vi "_FG_save_LV2018.vi"(6 "comment":string, 7 "error in":errorcluster, 8 "add EOL at end ?":bool, 9 "data in":variant, 10 "FG":T1) -> (0 "error IO":errorcluster={"status"=TRUE, "code"=1, "source"="Écrire dans un fichier texte dans _FG_save_LV2018.vi->save_all_parameters.vi->_main_program v5.vi"})   [LabVIEW 2018]
uses:
  enum_fg_save.ctl
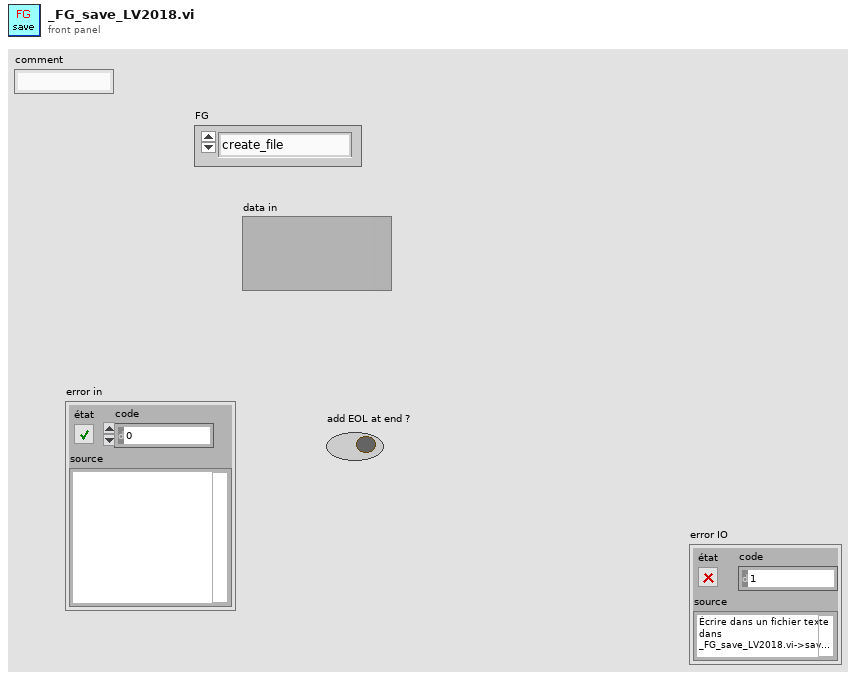
[diagram p1: front panel]
types:
  T1 = typedef "enum_fg_save.ctl" = enum16{"create_file", "w_array_text_inline", "w_text", "w_int", "w_uint", "w_single", "w_array", "w_array_inline", "w_clst_2arrays", "w_clst_3arrays", "w_clst_4arrays", "w_clst_5arrays", "w_clst_6arrays", "w_2Darray", "w_time", "close_file"}
  T2 = enum16{"open", "replace", "create", "open or create", "replace or create", "replace or create with confirmation"}
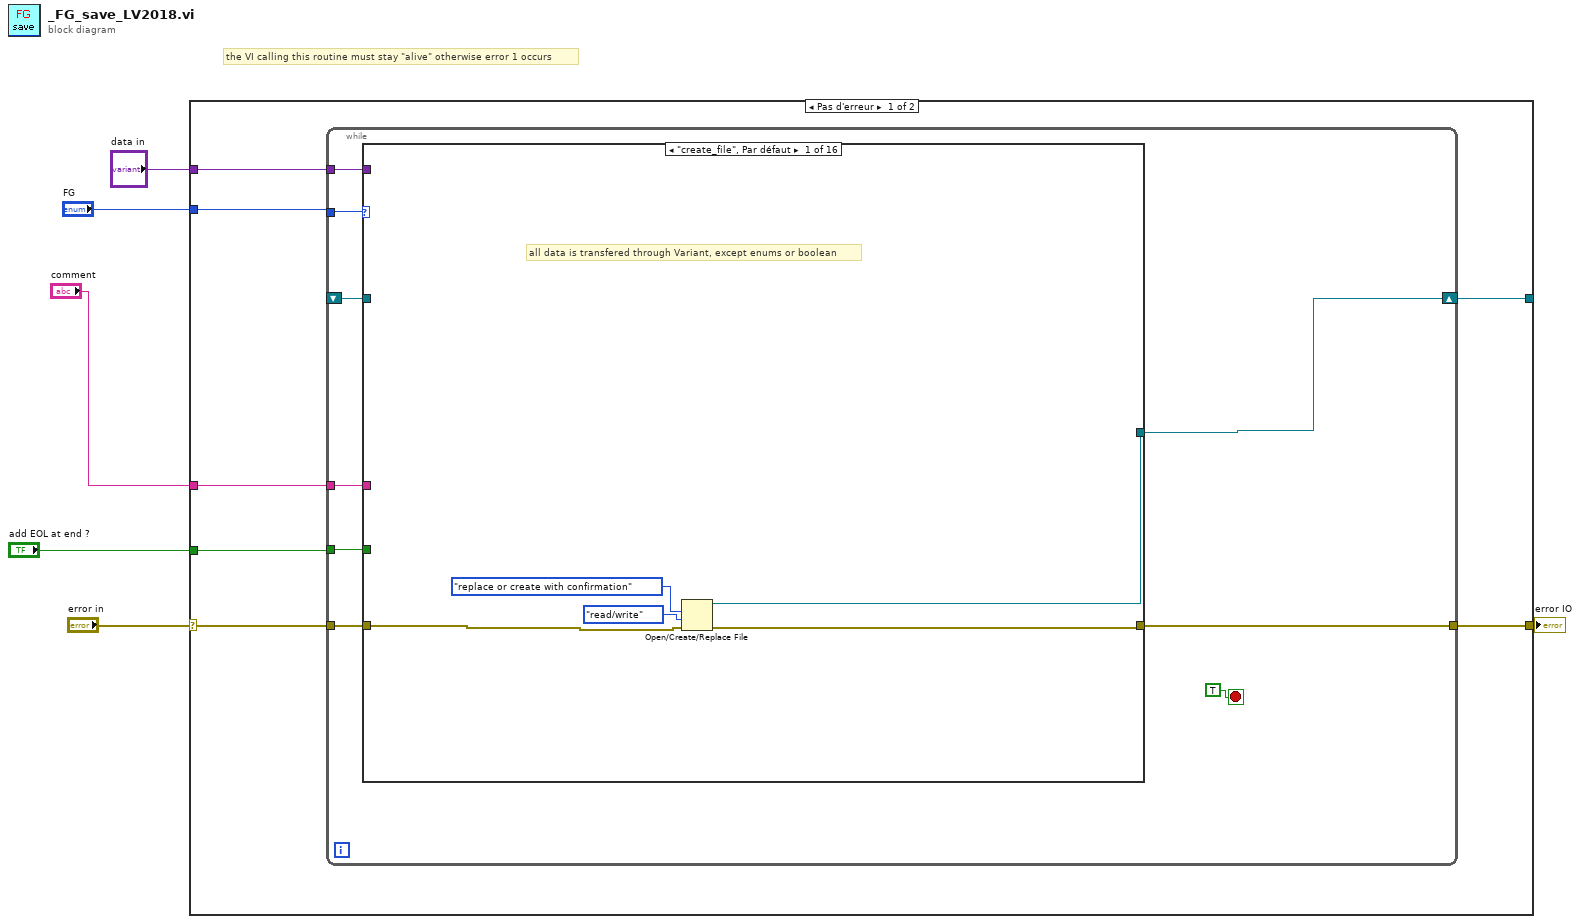
[diagram p0: block diagram]
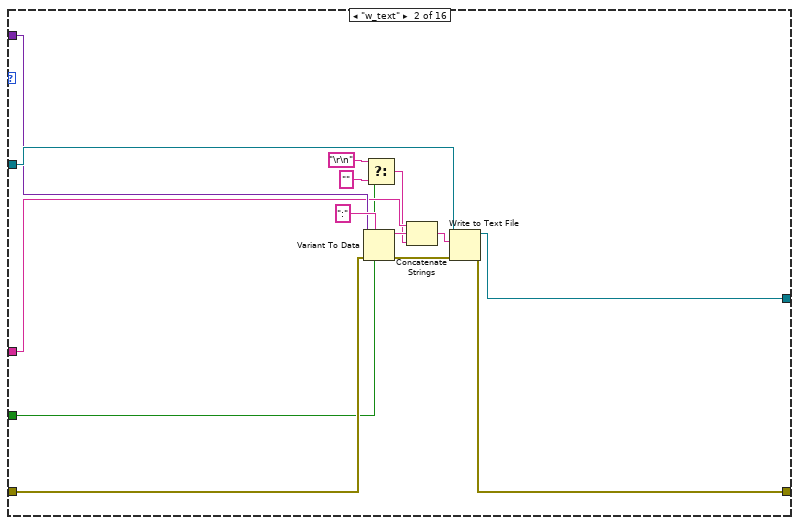
[diagram p2: hidden frame]
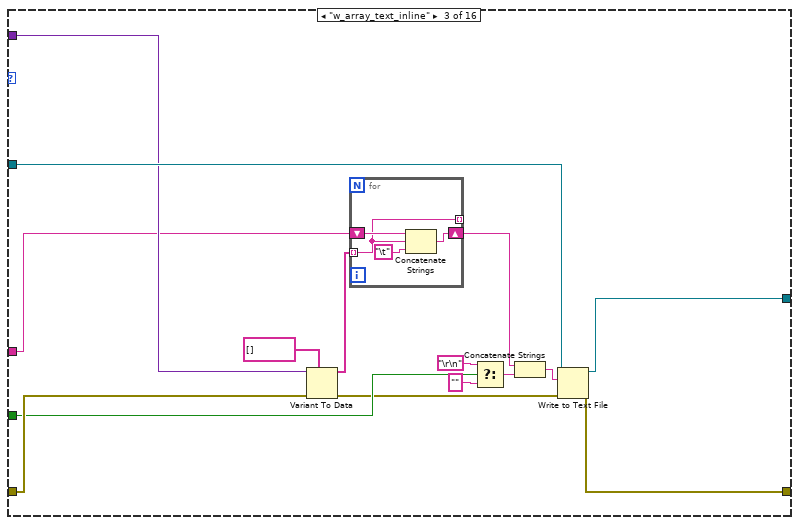
[diagram p3: hidden frame]
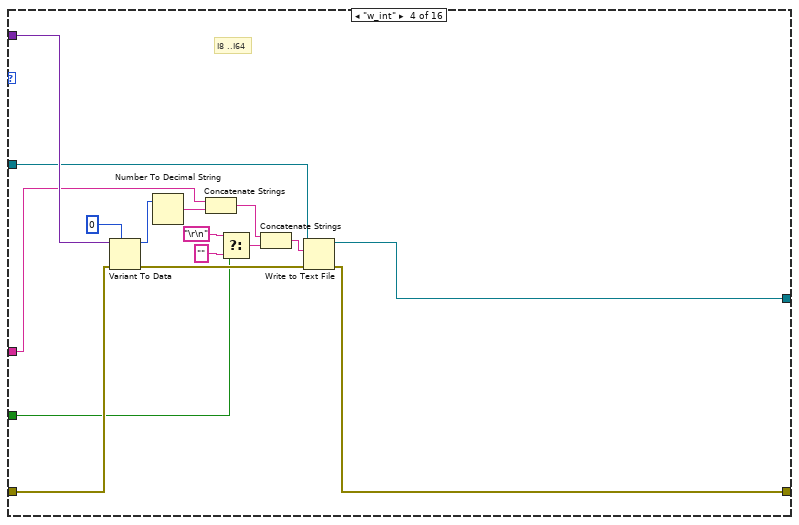
[diagram p4: hidden frame]
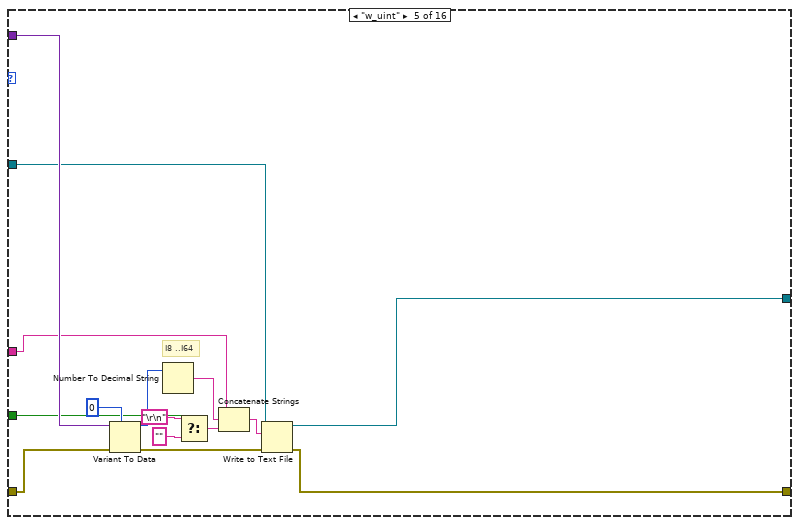
[diagram p5: hidden frame]
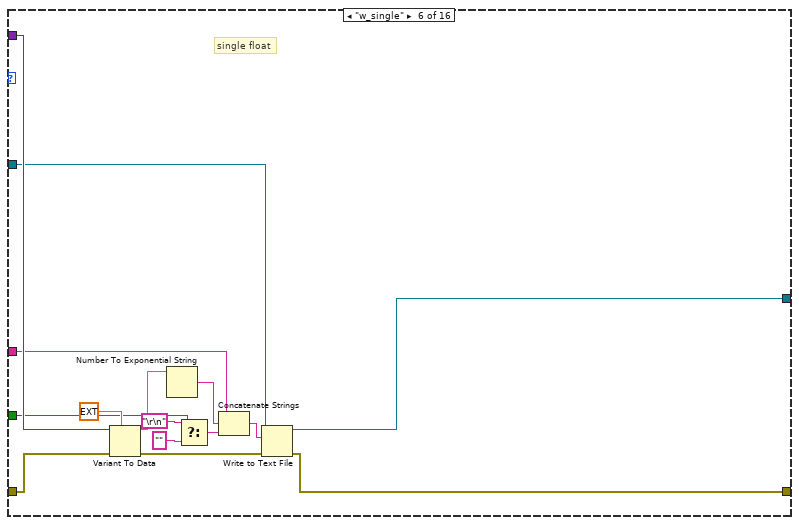
[diagram p6: hidden frame]
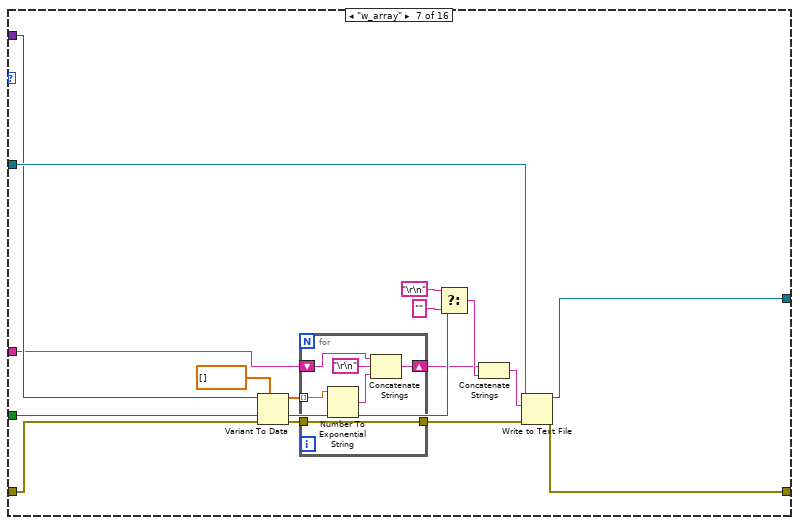
[diagram p7: hidden frame]
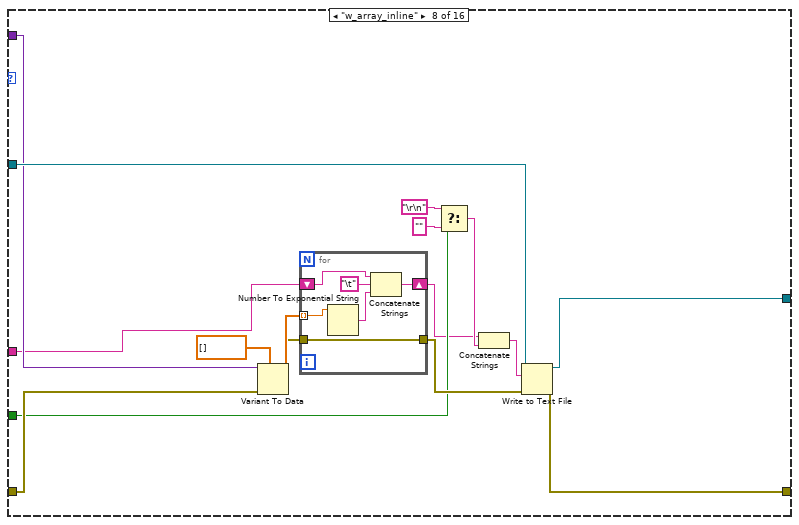
[diagram p8: hidden frame]
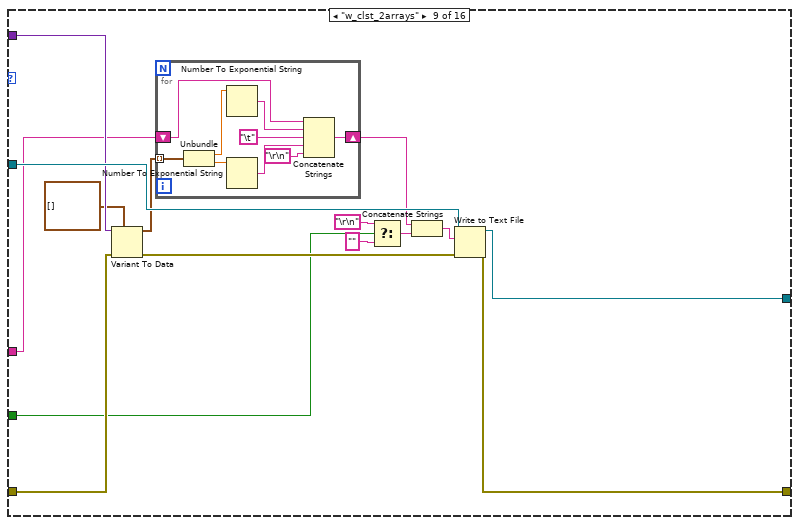
[diagram p9: hidden frame]
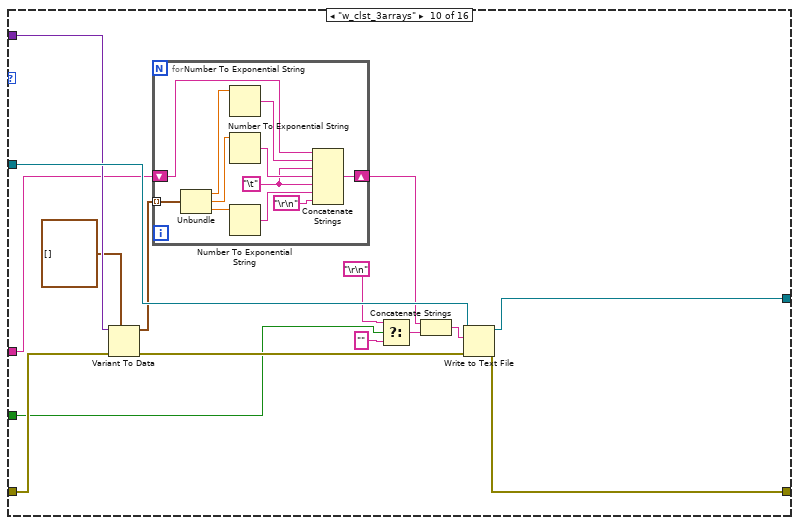
[diagram p10: hidden frame]
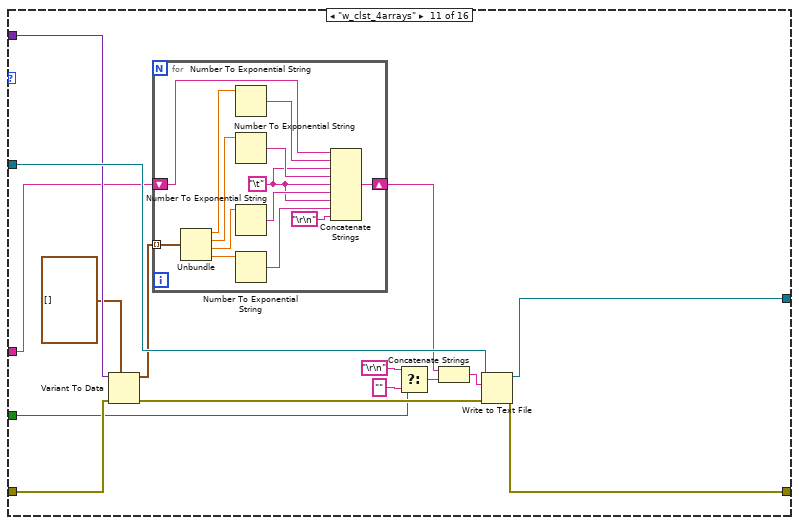
[diagram p11: hidden frame]
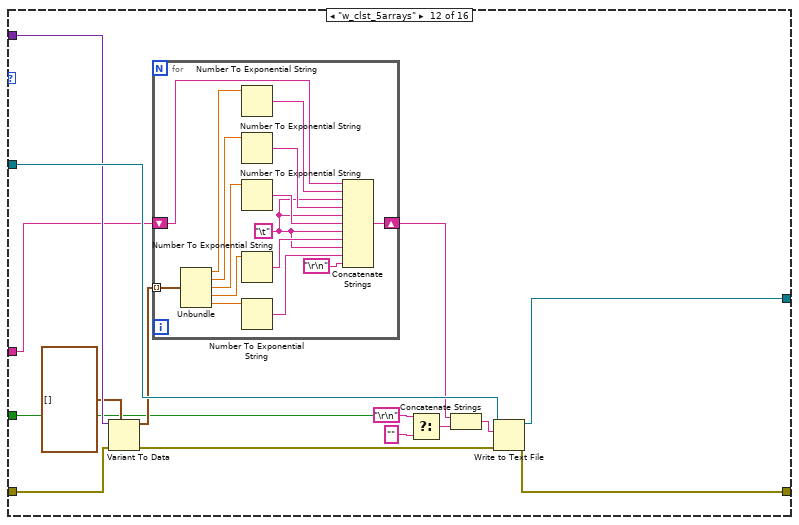
[diagram p12: hidden frame]
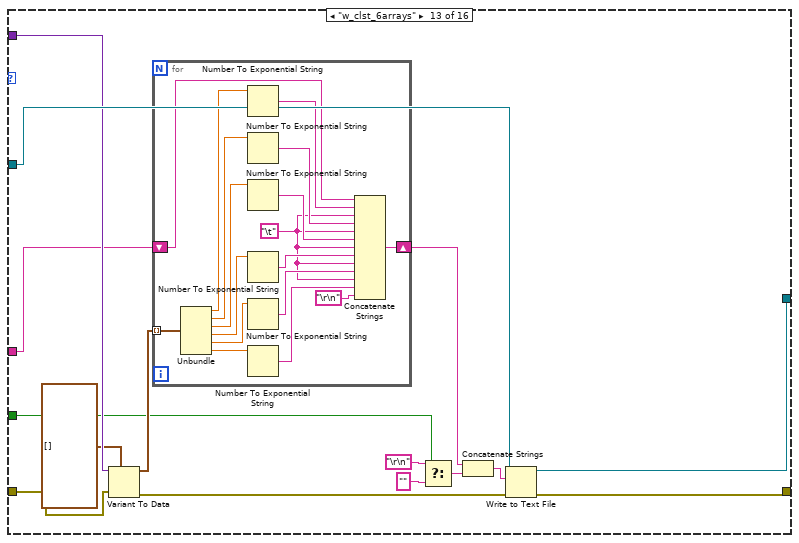
[diagram p13: hidden frame]
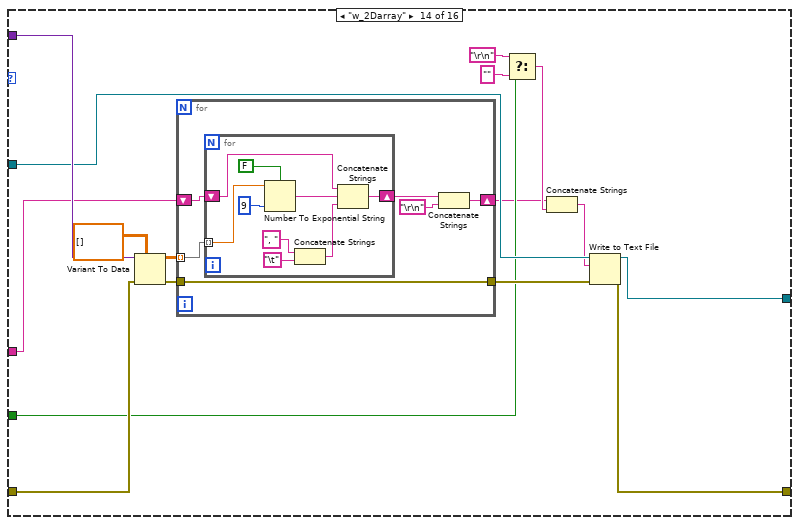
[diagram p14: hidden frame]
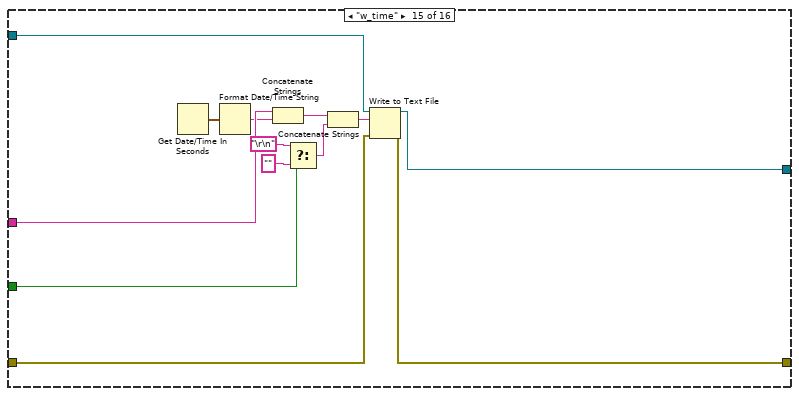
[diagram p15: hidden frame]
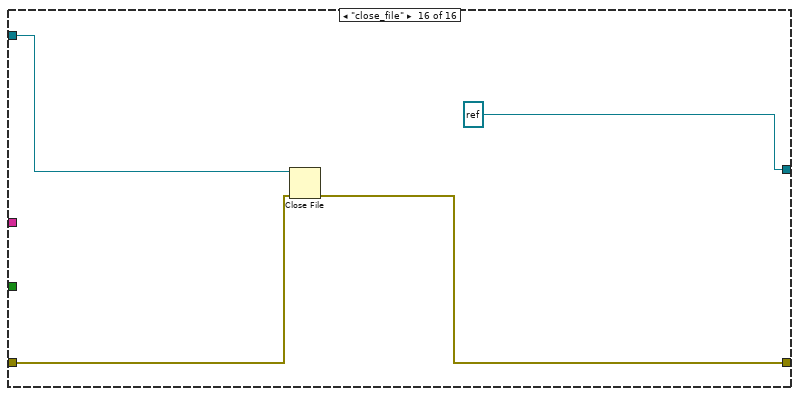
[diagram p16: hidden frame]
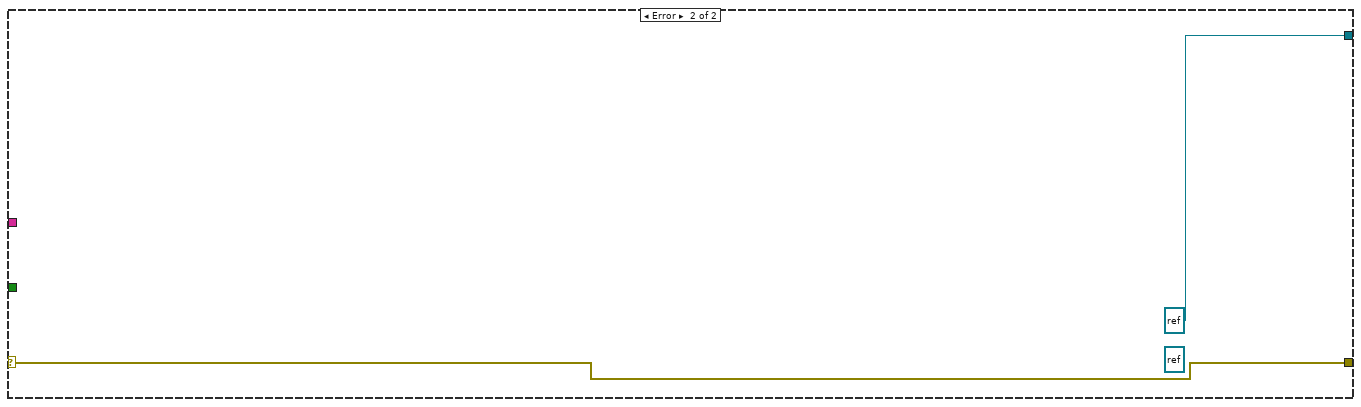
[diagram p17: hidden frame]
diagram:
  # "the VI calling this routine must stay \"alive\" otherwise error 1 occurs"
  n1 = case shown="Pas d'erreur" "error in" {
    selector: "error in" -> [w12 w339]
    tunnel: "FG" -> [w13 _]
    tunnel: [w11 refnum<file> refnum ("refnum out")] -> _
    tunnel: [w10 w339] -> w3
    tunnel: "data in" -> [w9 _]
    tunnel: "comment" -> [w8 _]
    tunnel: "add EOL at end ?" -> [w7 _]
    frame No Error {
      n2 = while {
        tunnel: w13 -> [w21]
        tunnel: w12 -> [w20]
        shift-right: [w15] -> w11
        shift-left: _ -> [w19]
        tunnel: [w14] -> w10
        tunnel: w9 -> [w18]
        tunnel: w8 -> [w17]
        tunnel: w7 -> [w16]
        stop <- TRUE stop-if-true
        n3 = case shown="\"create_file\", Par défaut" w21 {
          tunnel: w20 -> [w25 w36 w52 w74 w89 w104 w115 w137 w159 w183 w209 w237 w267 w304 w333 w335]
          tunnel: [w24 w40 w55 w71 w86 w101 w120 w142 w164 w188 w214 w242 w272 w299 w331 refnum<file> refnum ("refnum out")] -> w15
          tunnel: [w23 w41 w56 w70 w85 w100 w121 w143 w165 w189 w215 w243 w273 w300 w334 w336] -> w14
          tunnel: w19 -> [_ w39 w54 w72 w87 w102 w119 w141 w163 w187 w213 w241 w271 w298 w330 w338]
          tunnel: w18 -> [_ w37 w53 w75 w90 w105 w117 w139 w162 w186 w212 w240 w270 w305 _ _]
          tunnel: w17 -> [_ w35 w49 w68 w83 w98 w113 w135 w157 w181 w207 w235 w265 w297 w329 _]
          tunnel: w16 -> [_ w30 w44 w63 w78 w93 w109 w131 w153 w177 w203 w231 w261 w293 w324 _]
          frame "create_file", Default {
            # "all data is transfered through Variant, except enums or boolean"
            n4 = Open/Create/Replace File(error in=w25, operation (0:open)=T2."replace or create with confirmation" ("opération (0 : open)"), access (0:read/write)=enum16{"read/write", "read-only", "write-only"}."read/write" ("accès (0 : read/write)")) -> (refnum out=w24:refnum<file>, error out=w23:errorcluster)  [unwired: 3 in, 1 out]
          }
          frame "w_text" {
            n5 = Variant To Data(error in=w36, type=":" ("chaîne recherchée"), Variant=w37) -> (data=w34:string, error out=w28:errorcluster)
            n6 = Select(t="\r\n", s=w30, f="" ("cas faux")) -> (s? t:f=w29:string)
            n7 = Concatenate Strings(w35, w34, w29) -> (w33:string)
            n8 = Write to Text File(file (use dialog)=w39, text=w33, error in=w28) -> (refnum out=w40:refnum<file>, error out=w41:errorcluster)  [unwired: 1 in, 1 out]
          }
          frame "w_array_text_inline" {
            n9 = Variant To Data(error in=w52, type=string[] [] ("Tableau"), Variant=w53) -> (data=w50:string[], error out=w42:errorcluster)
            n10 = for {
              tunnel: [w59] -> _ mode=indexing
              tunnel: w50 -> [w59] mode=indexing
              shift-right: [w57] -> w46
              shift-left: w49 -> [w60]
              n11 = Concatenate Strings(w60, w59, "\t") -> (w57:string)
            }
            n12 = Select(t="\r\n", s=w44, f="" ("cas faux")) -> (s? t:f=w45:string)
            n13 = Concatenate Strings(w46, w45) -> (w43:string)
            n14 = Write to Text File(file (use dialog)=w54, text=w43, error in=w42) -> (refnum out=w55:refnum<file>, error out=w56:errorcluster)  [unwired: 1 in, 1 out]
          }
          frame "w_int" {
            # "I8 ..I64"
            n15 = Variant To Data(error in=w74, type=i64 0 ("r * e^(i*thêta)"), Variant=w75) -> (data=w73:i64, error out=w69:errorcluster)
            n16 = Number To Decimal String(number=w73) -> (decimal integer string=w67:string)  [unwired: 1 in]
            n17 = Concatenate Strings(w68, w67) -> (w62:string)
            n18 = Select(t="\r\n", s=w63, f="" ("cas faux")) -> (s? t:f=w64:string)
            n19 = Concatenate Strings(w62, w64) -> (w61:string)
            n20 = Write to Text File(file (use dialog)=w72, text=w61, error in=w69) -> (refnum out=w71:refnum<file>, error out=w70:errorcluster)  [unwired: 1 in, 1 out]
          }
          frame "w_uint" {
            # "I8 ..I64"
            n21 = Variant To Data(error in=w89, type=u64 0 ("r * e^(i*thêta)"), Variant=w90) -> (data=w88:u64, error out=w84:errorcluster)
            n22 = Number To Decimal String(number=w88) -> (decimal integer string=w82:string)  [unwired: 1 in]
            n23 = Select(t="\r\n", s=w78, f="" ("cas faux")) -> (s? t:f=w77:string)
            n24 = Concatenate Strings(w83, w82, w77) -> (w81:string)
            n25 = Write to Text File(file (use dialog)=w87, text=w81, error in=w84) -> (refnum out=w86:refnum<file>, error out=w85:errorcluster)  [unwired: 1 in, 1 out]
          }
          frame "w_single" {
            # "single float"
            n26 = Variant To Data(error in=w104, type=ext 0.0 ("r * e^(i*thêta)"), Variant=w105) -> (data=w103:ext, error out=w99:errorcluster)
            n27 = Number To Exponential String(number=w103) -> (E-format string=w97:string)  [unwired: 3 in]
            n28 = Select(t="\r\n", s=w93, f="" ("cas faux")) -> (s? t:f=w92:string)
            n29 = Concatenate Strings(w98, w97, w92) -> (w96:string)
            n30 = Write to Text File(file (use dialog)=w102, text=w96, error in=w99) -> (refnum out=w101:refnum<file>, error out=w100:errorcluster)  [unwired: 1 in, 1 out]
          }
          frame "w_array" {
            n31 = Variant To Data(error in=w115, type=dbl[] [] ("array 1"), Variant=w117) -> (data=w116:dbl[], error out=w114:errorcluster)
            n32 = for {
              tunnel: w116 -> [w127] mode=indexing
              shift-right: [w128] -> w108
              shift-left: w113 -> [w126]
              tunnel: w114 -> [w123]
              tunnel: [w123] -> w122
              n33 = Number To Exponential String(number=w127) -> (E-format string=w124:string)  [unwired: 3 in]
              n34 = Concatenate Strings(w126, "\r\n", w124) -> (w128:string)
            }
            n35 = Select(t="\r\n", s=w109, f="" ("cas faux")) -> (s? t:f=w110:string)
            n36 = Concatenate Strings(w108, w110) -> (w107:string)
            n37 = Write to Text File(file (use dialog)=w119, text=w107, error in=w122) -> (refnum out=w120:refnum<file>, error out=w121:errorcluster)  [unwired: 1 in, 1 out]
          }
          frame "w_array_inline" {
            n38 = Variant To Data(error in=w137, type=dbl[] [] ("array 1"), Variant=w139) -> (data=w138:dbl[], error out=w136:errorcluster)
            n39 = for {
              tunnel: w138 -> [w148] mode=indexing
              shift-right: [w149] -> w130
              shift-left: w135 -> [w147]
              tunnel: w136 -> [w150]
              tunnel: [w150] -> w144
              n40 = Number To Exponential String(number=w148) -> (E-format string=w145:string)  [unwired: 3 in]
              n41 = Concatenate Strings(w147, "\t", w145) -> (w149:string)
            }
            n42 = Select(t="\r\n", s=w131, f="" ("cas faux")) -> (s? t:f=w132:string)
            n43 = Concatenate Strings(w130, w132) -> (w129:string)
            n44 = Write to Text File(file (use dialog)=w141, text=w129, error in=w144) -> (refnum out=w142:refnum<file>, error out=w143:errorcluster)  [unwired: 1 in, 1 out]
          }
          frame "w_clst_2arrays" {
            n45 = Variant To Data(error in=w159, type=cluster{dbl, dbl}[] [] ("cluster of arrays"), Variant=w162) -> (data=w160:cluster{dbl, dbl}[], error out=w158:errorcluster)
            n46 = for {
              tunnel: w160 -> [w174] mode=indexing
              shift-right: [w173] -> w152
              shift-left: w157 -> [w172]
              n47 = Unbundle(w174) -> (w170:dbl, w168:dbl)
              n48 = Number To Exponential String(number=w170) -> (E-format string=w169:string)  [unwired: 3 in]
              n49 = Number To Exponential String(number=w168) -> (E-format string=w167:string)  [unwired: 3 in]
              n50 = Concatenate Strings(w172, w169, "\t", w167, "\r\n") -> (w173:string)
            }
            n51 = Select(t="\r\n", s=w153, f="" ("cas faux")) -> (s? t:f=w154:string)
            n52 = Concatenate Strings(w152, w154) -> (w151:string)
            n53 = Write to Text File(file (use dialog)=w163, text=w151, error in=w158) -> (refnum out=w164:refnum<file>, error out=w165:errorcluster)  [unwired: 1 in, 1 out]
          }
          frame "w_clst_3arrays" {
            n54 = Variant To Data(error in=w183, type=cluster{dbl, dbl, dbl}[] [] ("cluster of arrays"), Variant=w186) -> (data=w184:cluster{dbl, dbl, dbl}[], error out=w182:errorcluster)
            n55 = for {
              tunnel: w184 -> [w200] mode=indexing
              shift-right: [w199] -> w176
              shift-left: w181 -> [w198]
              w193 = "\t"
              n56 = Unbundle(w200) -> (w197:dbl, w195:dbl, w190:dbl)
              n57 = Number To Exponential String(number=w197) -> (E-format string=w196:string)  [unwired: 3 in]
              n58 = Number To Exponential String(number=w195) -> (E-format string=w194:string)  [unwired: 3 in]
              n59 = Number To Exponential String(number=w190) -> (E-format string=w192:string)  [unwired: 3 in]
              n60 = Concatenate Strings(w198, w196, w193, w194, w193, w192, "\r\n") -> (w199:string)
            }
            n61 = Select(t="\r\n", s=w177, f="" ("cas faux")) -> (s? t:f=w178:string)
            n62 = Concatenate Strings(w176, w178) -> (w175:string)
            n63 = Write to Text File(file (use dialog)=w187, text=w175, error in=w182) -> (refnum out=w188:refnum<file>, error out=w189:errorcluster)  [unwired: 1 in, 1 out]
          }
          frame "w_clst_4arrays" {
            n64 = Variant To Data(error in=w209, type=cluster{dbl, dbl, dbl, dbl}[] [] ("cluster of arrays"), Variant=w212) -> (data=w210:cluster{dbl, dbl, dbl, dbl}[], error out=w208:errorcluster)
            n65 = for {
              tunnel: w210 -> [w228] mode=indexing
              shift-right: [w227] -> w202
              shift-left: w207 -> [w226]
              w218 = "\t"
              n66 = Unbundle(w228) -> (w225:dbl, w223:dbl, w220:dbl, w217:dbl)
              n67 = Number To Exponential String(number=w225) -> (E-format string=w224:string)  [unwired: 3 in]
              n68 = Number To Exponential String(number=w223) -> (E-format string=w222:string)  [unwired: 3 in]
              n69 = Number To Exponential String(number=w220) -> (E-format string=w221:string)  [unwired: 3 in]
              n70 = Number To Exponential String(number=w217) -> (E-format string=w216:string)  [unwired: 3 in]
              n71 = Concatenate Strings(w226, w224, w218, w222, w218, w221, w218, w216, "\r\n") -> (w227:string)
            }
            n72 = Select(t="\r\n", s=w203, f="" ("cas faux")) -> (s? t:f=w204:string)
            n73 = Concatenate Strings(w202, w204) -> (w201:string)
            n74 = Write to Text File(file (use dialog)=w213, text=w201, error in=w208) -> (refnum out=w214:refnum<file>, error out=w215:errorcluster)  [unwired: 1 in, 1 out]
          }
          frame "w_clst_5arrays" {
            n75 = Variant To Data(error in=w237, type=cluster{dbl, dbl, dbl, dbl, dbl}[] [] ("cluster of arrays"), Variant=w240) -> (data=w238:cluster{dbl, dbl, dbl, dbl, dbl}[], error out=w236:errorcluster)
            n76 = for {
              tunnel: w238 -> [w258] mode=indexing
              shift-right: [w257] -> w230
              shift-left: w235 -> [w256]
              w246 = "\t"
              n77 = Unbundle(w258) -> (w255:dbl, w253:dbl, w250:dbl, w249:dbl, w245:dbl)
              n78 = Number To Exponential String(number=w255) -> (E-format string=w254:string)  [unwired: 3 in]
              n79 = Number To Exponential String(number=w253) -> (E-format string=w252:string)  [unwired: 3 in]
              n80 = Number To Exponential String(number=w250) -> (E-format string=w251:string)  [unwired: 3 in]
              n81 = Number To Exponential String(number=w249) -> (E-format string=w248:string)  [unwired: 3 in]
              n82 = Number To Exponential String(number=w245) -> (E-format string=w244:string)  [unwired: 3 in]
              n83 = Concatenate Strings(w256, w254, w246, w252, w246, w251, w246, w248, w246, w244, "\r\n") -> (w257:string)
            }
            n84 = Select(t="\r\n", s=w231, f="" ("cas faux")) -> (s? t:f=w232:string)
            n85 = Concatenate Strings(w230, w232) -> (w229:string)
            n86 = Write to Text File(file (use dialog)=w241, text=w229, error in=w236) -> (refnum out=w242:refnum<file>, error out=w243:errorcluster)  [unwired: 1 in, 1 out]
          }
          frame "w_clst_6arrays" {
            n87 = Variant To Data(error in=w267, type=cluster{dbl, dbl, dbl, dbl, dbl, dbl}[] [] ("cluster of arrays"), Variant=w270) -> (data=w268:cluster{dbl, dbl, dbl, dbl, dbl, dbl}[], error out=w266:errorcluster)
            n88 = for {
              tunnel: w268 -> [w290] mode=indexing
              shift-right: [w289] -> w260
              shift-left: w265 -> [w288]
              w277 = "\t"
              n89 = Unbundle(w290) -> (w287:dbl, w285:dbl, w282:dbl, w281:dbl, w279:dbl, w276:dbl)
              n90 = Number To Exponential String(number=w287) -> (E-format string=w286:string)  [unwired: 3 in]
              n91 = Number To Exponential String(number=w285) -> (E-format string=w284:string)  [unwired: 3 in]
              n92 = Number To Exponential String(number=w282) -> (E-format string=w283:string)  [unwired: 3 in]
              n93 = Number To Exponential String(number=w281) -> (E-format string=w280:string)  [unwired: 3 in]
              n94 = Number To Exponential String(number=w279) -> (E-format string=w278:string)  [unwired: 3 in]
              n95 = Number To Exponential String(number=w276) -> (E-format string=w275:string)  [unwired: 3 in]
              n96 = Concatenate Strings(w288, w286, w277, w284, w277, w283, w277, w280, w277, w278, w277, w275, "\r\n") -> (w289:string)
            }
            n97 = Select(t="\r\n", s=w261, f="" ("cas faux")) -> (s? t:f=w262:string)
            n98 = Concatenate Strings(w260, w262) -> (w259:string)
            n99 = Write to Text File(file (use dialog)=w271, text=w259, error in=w266) -> (refnum out=w272:refnum<file>, error out=w273:errorcluster)  [unwired: 1 in, 1 out]
          }
          frame "w_2Darray" {
            n100 = Variant To Data(error in=w304, type=sgl[][] [] ("tableau ajouté"), Variant=w305) -> (data=w303:sgl[][], error out=w302:errorcluster)
            n101 = for {
              tunnel: w303 -> [w312] mode=indexing
              shift-right: [w308] -> w292
              shift-left: w297 -> [w311]
              tunnel: [w307] -> w301
              tunnel: w302 -> [w307]
              n102 = for {
                tunnel: w312 -> [w321] mode=indexing
                shift-right: [w319] -> w309
                shift-left: w311 -> [w318]
                n103 = Number To Exponential String(number=w321, precision (6)=i16 9 ("précision (6)"), 1:FALSE ("utiliser le séparateur décimal du système (V)")) -> (E-format string=w320:string)  [unwired: 1 in]
                n104 = Concatenate Strings(", " ("chaîne"), "\t") -> (w313:string)
                n105 = Concatenate Strings(w318, w320, w313) -> (w319:string)
              }
              n106 = Concatenate Strings(w309, "\r\n") -> (w308:string)
            }
            n107 = Select(t="\r\n", s=w293, f="" ("cas faux")) -> (s? t:f=w294:string)
            n108 = Concatenate Strings(w292, w294) -> (w291:string)
            n109 = Write to Text File(file (use dialog)=w298, text=w291, error in=w301) -> (refnum out=w299:refnum<file>, error out=w300:errorcluster)  [unwired: 1 in, 1 out]
          }
          frame "w_time" {
            n110 = Get Date/Time In Seconds() -> (seconds since 1Jan1904=w332:timestamp)
            n111 = Format Date/Time String(seconds (now)=w332) -> (date/time string=w328:string)  [unwired: 2 in]
            n112 = Concatenate Strings(w329, w328) -> (w323:string)
            n113 = Select(t="\r\n", s=w324, f="" ("cas faux")) -> (s? t:f=w325:string)
            n114 = Concatenate Strings(w323, w325) -> (w322:string)
            n115 = Write to Text File(file (use dialog)=w330, text=w322, error in=w333) -> (refnum out=w331:refnum<file>, error out=w334:errorcluster)  [unwired: 1 in, 1 out]
          }
          frame "close_file" {
            n116 = Close File(refnum=w338, error in=w335) -> (error out=w336:errorcluster)  [unwired: 1 out]
          }
        }
      }
    }
    frame Error {
      (unwired) refnum<file> refnum ("refnum out")
    }
  }
  "error IO" <- w3
